vi "GUI PS Group Indexes.vi"(11 "PS Group":enum16{"ACH", "ACV", "ALV"}(ring)) -> (3 "Indexes":i32[](array[numeric]))   [LabVIEW 2011, in "User Interface VIs.lvlib"]
uses:
  User Interface VIs.lvlib
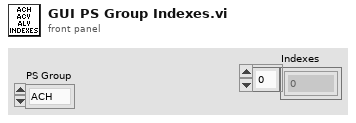
[diagram p1: front panel]
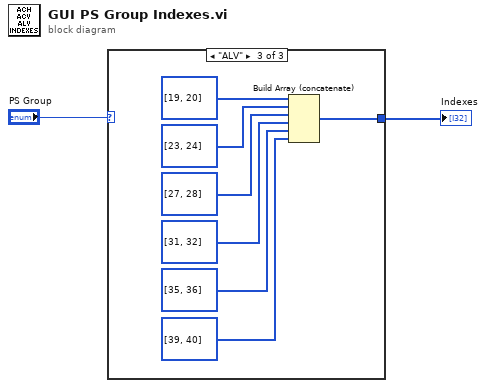
[diagram p0: block diagram]
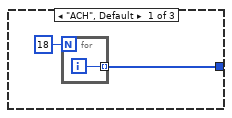
[diagram p2: hidden frame]
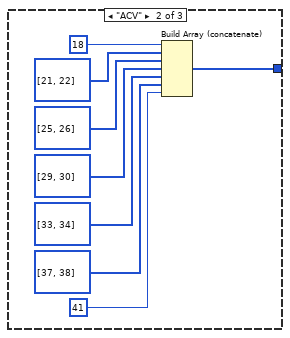
[diagram p3: hidden frame]
diagram:
  n1 = case shown="\"ALV\"" "PS Group" {
    tunnel: [w3 w6 w14] -> w2
    frame "ACH", Default {
      n2 = for {
        N: 18 -> [_]
        tunnel: [w5] -> w3 mode=indexing
        i -> [w5]
      }
    }
    frame "ACV" {
      n3 = Build Array (concatenate)(18 ("index"), i32[] [21, 22], i32[] [25, 26], i32[] [29, 30], i32[] [33, 34], i32[] [37, 38], 41 ("index")) -> (w6:i32[])
    }
    frame "ALV" {
      n4 = Build Array (concatenate)(i32[] [19, 20], i32[] [23, 24], i32[] [27, 28], i32[] [31, 32], i32[] [35, 36], i32[] [39, 40]) -> (w14:i32[])
    }
  }
  "Indexes" <- w2
